vi "Copy_Settings.vi"(8 "error in (no error)":errorcluster, 10 "LabVIEW Object":refnum<class>, 11 "IB_Settings_Item_Destination in":refnum<class "IB_Settings_Item_Destination.lvclass">) -> (0 "error out":errorcluster, 3 "IB_Settings_Item_Destination out":refnum<class "IB_Settings_Item_Destination.lvclass">)   [LabVIEW 2020, in "IB_Settings_Item_Destination.lvclass"]
uses:
  <vilib>/AppBuilder/IB_Classes/Settings_Item_Destination/IB_Settings_Item_Destination.lvclass
  <vilib>/AppBuilder/IB_Classes/Settings_Item_Destination/IB_Settings_Item_Destination.lvclass/IB_Settings_Item_Destination.ctl
  <vilib>/AppBuilder/IB_Classes/Destination/IB_Destination.lvclass
  <vilib>/AppBuilder/IB_Classes/Settings_Item/IB_Settings_Item.lvclass
  e:/builds/penguin/labview/branches/2020/dev/dist/vi.lib/AppBuilder/IB_Classes/Settings_Item/IB_Settings_Item.lvclass
  e:/builds/penguin/labview/branches/2020/dev/dist/vi.lib/AppBuilder/IB_Classes/Settings_Item_Destination/IB_Settings_Item_Destination.lvclass
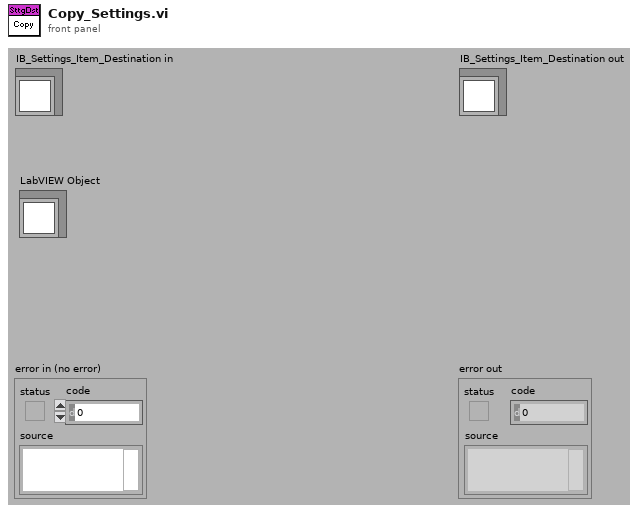
[diagram p1: front panel]
types:
  T1 = typedef "IB_Destination.ctl" = cluster{"name":string, "unlock":bool, "parentTag":string, "destTag":string, "eng_installPath":string}
  T2 = typedef "IB_Settings_Item.ctl" = cluster{"address":string[], "Attributes":i16, "RegCOM":bool, "unlock":bool}
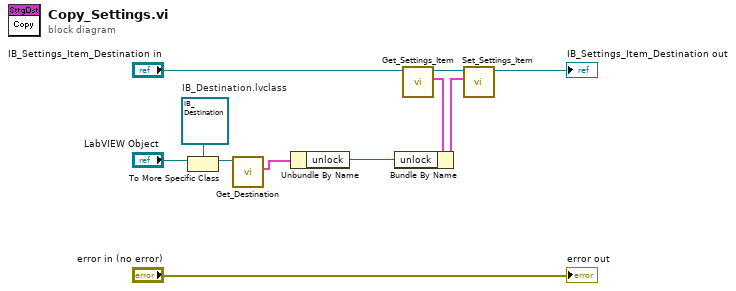
[diagram p0: block diagram]
diagram:
  w10 = refnum<class "IB_Destination.lvclass"> refnum  # IB_Destination.lvclass
  n1 = To More Specific Class(target class=w10, reference="LabVIEW Object") -> (specific class reference=w4:refnum<class "IB_Destination.lvclass">)  [unwired: 1 in, 1 out]
  n2 = call <vilib>:"Get_Destination.vi"("IB_Destination in"=w4) -> ("data"=w3:T1)  [unwired: 8 in, 2 out]
  n3 = Unbundle By Name(w3) -> ("unlock"=w2:bool)
  n4 = call <vilib>:"Get_Settings_Item.vi"("IB_Settings_Item in"="IB_Settings_Item_Destination in") -> ("data"=w6:T2, "IB_Settings_Item out"=w7:refnum<class "IB_Settings_Item_Destination.lvclass">)  [unwired: 8 in, 1 out]
  n5 = Bundle By Name(cluster=w6, "unlock"=w2) -> (w5:T2)
  n6 = call <vilib>:"Set_Settings_Item.vi"("data"=w5, "IB_Settings_Item in"=w7) -> ("IB_Settings_Item out"=→"IB_Settings_Item_Destination out":refnum<class "IB_Settings_Item_Destination.lvclass">)  [unwired: 8 in, 1 out]
  "error out" <- "error in (no error)"
